vi "IMAQ FPGA CXP Data to Vision Pixel Bus 8-Bit x 8.vi"(7 "Reset":bool, 10 "Image Size":cluster{"Width":u16, "Height":u16}, 11 "CXP Data":T1) -> (0 "EOI":bool, 1 "EOL":bool, 2 "DV":bool[](array[boolean]), 3 "Pixel Data":u8[](array[numeric]), 4 "Ready for Input":bool)   [LabVIEW 2020]
uses:
  <vilib>/visionFPGA/Basics/CoaXPress Acquisition/Controls/IMAQ FPGA CXP NI AXI4-S Bus.ctl
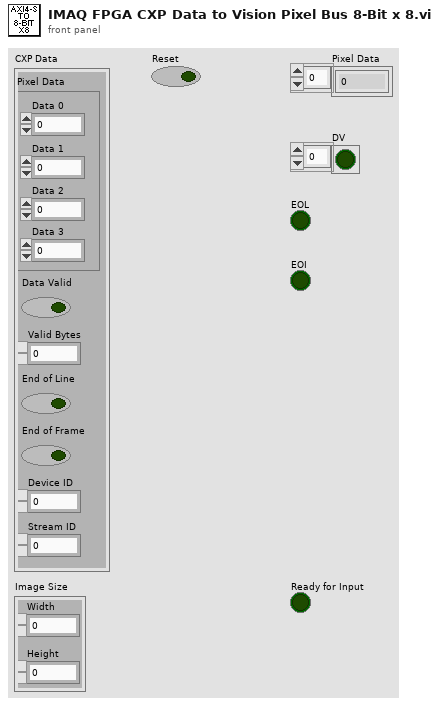
[diagram p1: front panel]
types:
  T1 = typedef "IMAQ FPGA CXP NI AXI4-S Bus.ctl" = cluster{"Pixel Data":cluster{"Data 0":u64, "Data 1":u64, "Data 2":u64, "Data 3":u64}, "Data Valid":bool, "Valid Bytes":u8, "End of Line":bool, "End of Frame":bool, "Device ID":u8, "Stream ID":u8}
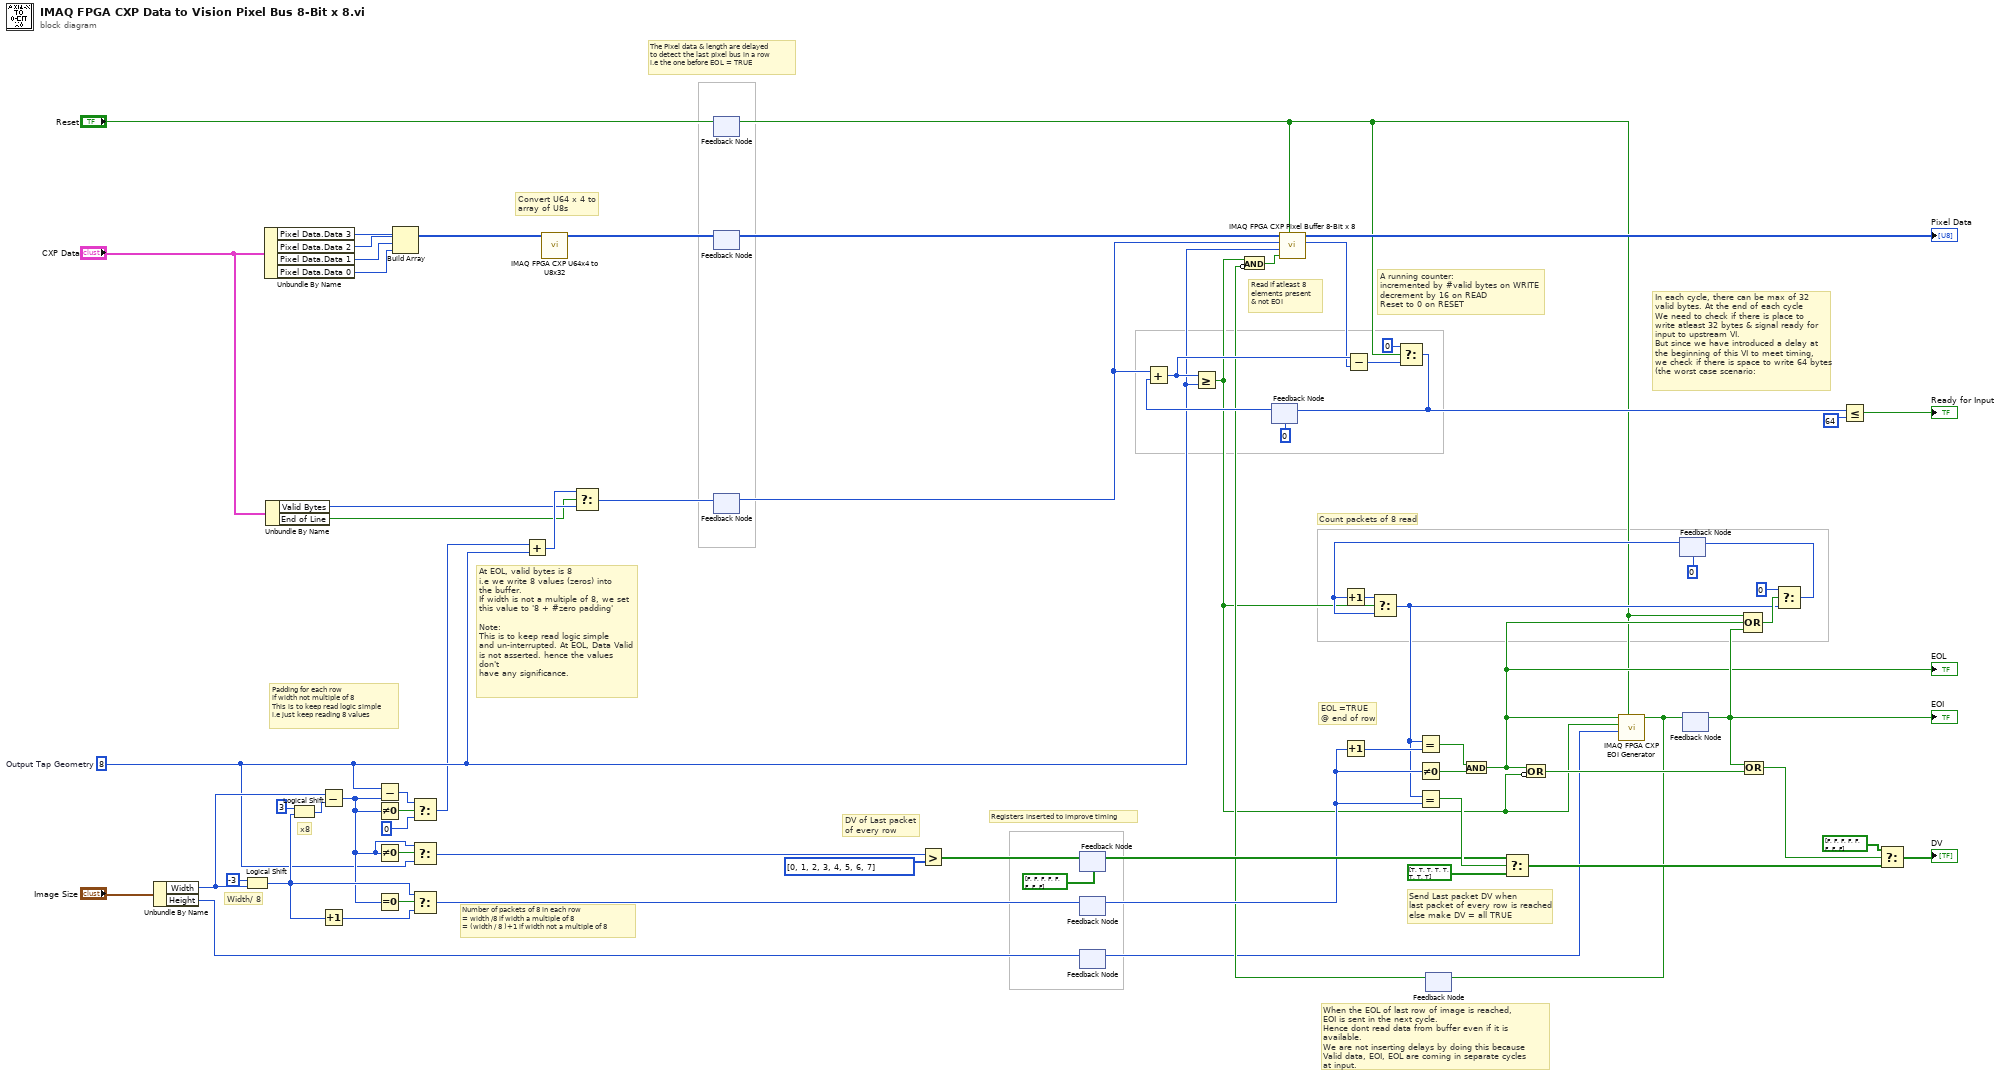
[diagram p0: block diagram]
diagram:
  w15 = u8 8  # Output Tap Geometry
  # "A running counter:\nincremented by #valid bytes on WRITE\ndecrement by 16 on READ\nReset to 0 on RESET"
  # "Padding for each row\nif width not multiple of 8\nThis is to keep read logic simple\ni.e just keep reading 8 values"
  # "x8"
  # "Width/ 8"
  # "When the EOL of last row of image is reached,\nEOI is sent in the next cycle. \nHence dont read data from buffer even if it is available.\nWe are not inserting delays by doing this because \nValid data, EOI, EOL are coming in separate cycles\nat input."
  # "EOL =TRUE\n@ end of row"
  # "Count packets of 8 read"
  # "Send Last packet DV when\nlast packet of every row is reached\nelse make DV = all TRUE"
  # "Convert U64 x 4 to \narray of U8s"
  # "In each cycle, there can be max of 32\nvalid bytes. At the end of each cycle\nWe need to check if there is place to \nwrite atleast 32 bytes & signal ready for\ninput to upstream VI.\nBut since we have introduced a delay at\nthe beginning of this VI to meet timing,\nwe check if there is space to write 64 bytes\n(the worst case scenario:"
  # "Read if atleast 8\nelements present\n& not EOI"
  # "Number of packets of 8 in each row\n= width /8 if width a multiple of 8\n= (width / 8 )+1 if width not a multiple of 8"
  # "DV of Last packet \nof every row"
  # "At EOL, valid bytes is 8\ni.e we write 8 values (zeros) into\nthe buffer.\nIf width is not a multiple of 8, we set\nthis value to '8 + #zero padding'\n\nNote:\nThis is to keep read logic simple\nand un-interrupted. At EOL, Data Valid\nis not asserted. hence the values don't\nhave any significance."
  # "Registers inserted to improve timing"
  # "The Pixel data & length are delayed\nto detect the last pixel bus in a row\ni.e the one before EOL = TRUE"
  n1 = Unbundle By Name("Image Size") -> ("Width"=w42:u16, "Height"=w34:u16)
  n2 = Logical Shift(y=i16 -3, x=w42) -> (x << y=w52:u16)
  n3 = Unbundle By Name("CXP Data") -> ("Pixel Data.Data 3"=w23:u64, "Pixel Data.Data 2"=w22:u64, "Pixel Data.Data 1"=w21:u64, "Pixel Data.Data 0"=w20:u64)
  n4 = Unbundle By Name("CXP Data") -> ("Valid Bytes"=w24:u8, "End of Line"=w19:bool)
  n5 = Logical Shift(y=i16 3, x=w52) -> (x << y=w48:u16)
  n6 = Subtract(x=w42, y=w48) -> (x-y=w46:u16)
  n7 = Increment(x=w52) -> (x+1=w64:u16)
  n8 = Subtract(x=w15, y=w46) -> (x-y=w49:u8)
  n9 = Not Equal To 0?(x=w46) -> (x != 0?=w50:bool)
  n10 = Not Equal To 0?(x=w46) -> (x != 0?=w47:bool)
  n11 = Equal To 0?(x=w46) -> (x = 0?=w65:bool)
  n12 = Build Array(w23, w22, w21, w20) -> (w57:u64[])
  n13 = Select(t=w49, s=w50, f=u8 0 ("x")) -> (s? t:f=w10:u8)
  n14 = Select(t=w46, s=w47, f=w15) -> (s? t:f=w45:u16)
  n15 = Select(t=w52, s=w65, f=w64) -> (s? t:f=w35:u16)
  n16 = Add(x=w10, y=w15) -> (x+y=w30:u8)
  n17 = call <vilib>:"IMAQ FPGA CXP U64x4 to U8x32.vi"("Pixel Data U64x4"=w57) -> ("Pixel Data Out U8x32"=w26:u8[])  [unwired: 10 in]
  n18 = Select(t=w30, s=w19, f=w24) -> (s? t:f=w56:u8)
  n19 = feedback #1() -> (w1:bool)  [unwired: 1 in]
  n20 = feedback-in #1("Reset") -> ()
  n21 = feedback-in #2(w26) -> ()
  n22 = feedback #2() -> (w13:u8[])  [unwired: 1 in]
  n23 = feedback-in #3(w56) -> ()
  n24 = feedback #3() -> (w14:u8)  [unwired: 1 in]
  n25 = Greater?(x=w45, y=u16[] [0, 1, 2, 3, 4, 5, 6, 7]) -> (0:w37:bool[])
  n26 = feedback #4(bool[] [FALSE, FALSE, FALSE, FALSE, FALSE, FALSE, FALSE, FALSE] ("x > y?")) -> (w36:bool[])
  n27 = feedback-in #4(w37) -> ()
  n28 = feedback #5() -> (w28:u16)  [unwired: 1 in]
  n29 = feedback-in #5(w35) -> ()
  n30 = feedback #6() -> (w3:u16)  [unwired: 1 in]
  n31 = feedback-in #6(w34) -> ()
  n32 = feedback #7(u8 0) -> (w71:u8)
  n33 = Add(x=w14, y=w71) -> (x+y=w70:u8)
  n34 = Greater Or Equal?(x=w70, y=w15) -> (x >= y?=w4:bool)
  n35 = Increment(x=w28) -> (x+1=w29:u16)
  n36 = Not Equal To 0?(x=w28) -> (x != 0?=w31:bool)
  n37 = feedback #8() -> (w11:bool)  [unwired: 1 in]
  n38 = Compound Arithmetic op=AND(w4, invert w11) -> (w12:bool)
  n39 = call <vilib>:"IMAQ FPGA CXP Pixel Buffer 8-Bit x 8.vi"("Reset"=w1, "Read"=w12, "Tap"=w15, "Valid Bytes"=w14, "Pixel Data In U8x32"=w13) -> ("#Elements Read"=w16:u8, "Pixel Data Out U8x8"=→"Pixel Data":u8[])  [unwired: 5 in]
  n40 = Subtract(x=w70, y=w16) -> (x-y=w8:u8)
  n41 = Select(t=u8 0, s=w1, f=w8) -> (s? t:f=w7:u8)
  n42 = feedback-in #7(w7) -> ()
  n43 = feedback #9(u16 0) -> (w44:u16)
  n44 = Increment(x=w44) -> (x+1=w62:u16)
  n45 = Select(t=w62, s=w4, f=w44) -> (s? t:f=w27:u16)
  n46 = Equal?(x=w27, y=w29) -> (x = y?=w32:bool)
  n47 = Equal?(x=w27, y=w28) -> (x = y?=w61:bool)
  n48 = And(x=w32, y=w31) -> (x .and. y?=w2:bool)
  "EOL" <- w2
  n49 = Select(t=w36, s=w61, f=bool[] [TRUE, TRUE, TRUE, TRUE, TRUE, TRUE, TRUE, TRUE] ("x > y?")) -> (s? t:f=w59:bool[])
  n50 = Compound Arithmetic op=OR(w2, invert w4) -> (w41:bool)
  n51 = call <vilib>:"IMAQ FPGA CXP EOI Generator.vi"("Reset"=w1, "Height"=w3, "Enable"=w4, "EOL"=w2) -> ("EOI"=w5:bool)  [unwired: 7 in]
  n52 = feedback-in #8(w5) -> ()
  n53 = feedback-in #10(w5) -> ()
  n54 = feedback #10() -> (w38:bool)  [unwired: 1 in]
  "EOI" <- w38
  n55 = Compound Arithmetic op=OR(w1, w2, w38) -> (w39:bool)
  n56 = Compound Arithmetic op=OR(w38, w41) -> (w40:bool)
  n57 = Select(t=u16 0, s=w39, f=w27) -> (s? t:f=w55:u16)
  n58 = feedback-in #9(w55) -> ()
  n59 = Less Or Equal?(x=w7, y=u8 64) -> (x <= y?=→"Ready for Input":bool)
  n60 = Select(t=bool[] [FALSE, FALSE, FALSE, FALSE, FALSE, FALSE, FALSE, FALSE] ("x > y?"), s=w40, f=w59) -> (s? t:f=→"DV":bool[])
